vi "DrawJoint.vi"(2 "Start":T1=[[1.0, 0.0, 0.0, 0.0], [0.0, 1.0, 0.0, 0.0], [0.0, 0.0, 1.0, 0.0], [0.0, 0.0, 0.0, 1.0]], 3 "Stage in":refnum<vi>) -> (1 "Stage out":refnum<vi>)   [LabVIEW 2024]
uses:
  <vilib>/Analysis/Matrix/Datatypes/RealMatrix.ctl
  <vilib>/picture/3D Picture Control/NI_3D Picture Control.lvlib
  <vilib>/robotics/Kinematics/NI_Kinematics.lvlib
  <vilib>/Analysis/Matrix/NI_Matrix.lvlib
panel:
  out "error out":errorcluster
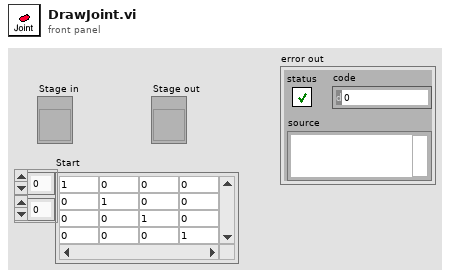
[diagram p1: front panel]
types:
  T1 = typedef "NI_Matrix.lvlib/RealMatrix.ctl" = dbl[][]
  T2 = cluster{"Height":sgl, "Radius":sgl, "Color Box":u32, "Alpha":sgl, "Detail":sgl}
  T3 = cluster{"Position[0]":dbl, "Position[1]":dbl, "Position[2]":dbl}
  T4 = cluster{"vector[0]":dbl, "vector[1]":dbl, "vector[2]":dbl}
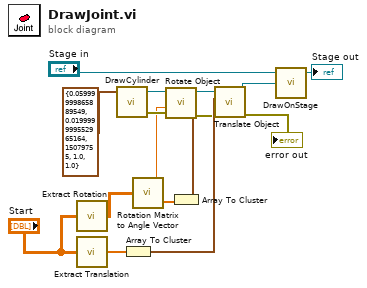
[diagram p0: block diagram]
diagram:
  n1 = call <userlib>:"Extract Rotation.vi"("Transformation matrix"="Start") -> ("Rotation matrix"=w4:T1)
  n2 = call <userlib>:"Extract Translation.vi"("Transformation matrix"="Start") -> ("Position"=w6:dbl[])
  n3 = call <userlib>:"DrawCylinder.vi"("Cylinder"=T2 {"Height"=0.06, "Radius"=0.02, "Color Box"=15079755, "Alpha"=1.0, "Detail"=1.0}) -> ("object out"=w9:refnum<vi>, "error out"=w7:errorcluster)  [unwired: 5 in]
  n4 = Array To Cluster(array=w6) -> (cluster=w12:T3)
  n5 = call <vilib>:"Rotation Matrix to Angle Vector.vi"("rotation matrix"=w4) -> ("angle"=w3:dbl, "vector"=w2:dbl[])
  n6 = Array To Cluster(array=w2) -> (cluster=w1:T4)
  n7 = call <vilib>:"Rotate Object.vi"("error in (no error)"=w7, "Angle"=w3, "Axis"=w1, "Scene.Object In"=w9) -> ("error out"=w10:errorcluster, "Scene.Object Out"=w8:refnum<vi>)  [unwired: 6 in]
  n8 = call <vilib>:"Translate Object.vi"("error in (no error)"=w10, "Translation"=w12, "Scene.Object In"=w8) -> ("error out"=→"error out":errorcluster, "Scene.Object Out"=w13:refnum<vi>)  [unwired: 7 in]
  n9 = call <userlib>:"DrawOnStage.vi"("object in"=w13, "Stage in"="Stage in") -> ("Stage out"=→"Stage out":refnum<vi>)  [unwired: 1 in, 2 out]
